vi "Finite Sound Input.vi"() -> ()   [LabVIEW 2023]
doc: "This VI illustrates how to acquire a finite number of samples from a specified device. It requires the use of a microphone attached to the sound card. You can specify the number of samples to acquire, sample rate, number of channels and a bit rate per sample."
uses:
  <vilib>/sound2/lvsound2.llb/Sampling Mode.ctl
  <vilib>/sound2/lvsound2.llb/Sound Data Format.ctl
  <vilib>/sound2/lvsound2.llb/Sound Input Read (DBL).vi
panel:
  in  "Device ID":u32
  out "Sound Input":waveform(dbl)[](graph)
  in  "Number of Samples/ch":i32=10000
  # "Overview: Demonstrates the use of the Sound Functions to acquire a finite number of samples from a microphone attached to the sound card.\nRequirements: Microphone\nInstructions:\n1. Specify the Device ID and Number of Samples/ch.\n2. Run the VI."
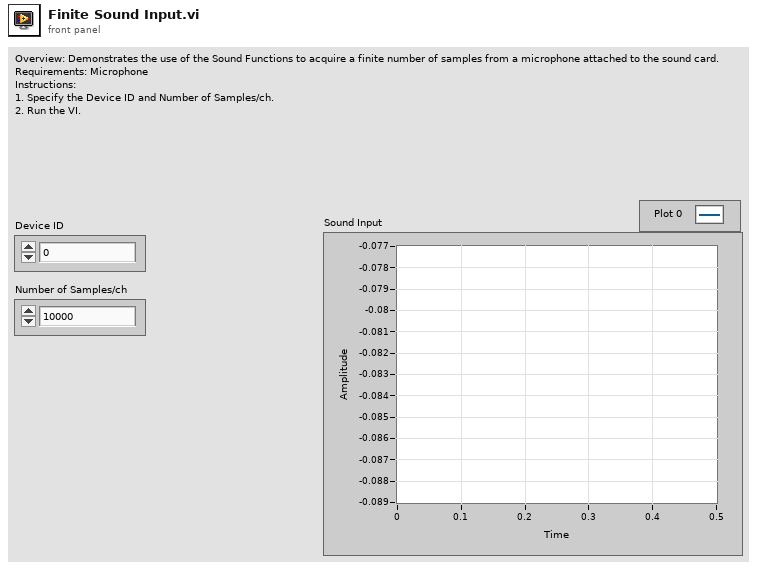
[diagram p1: front panel]
types:
  T1 = typedef "Sound Data Format.ctl" = cluster{"sample rate (S/s)":dbl, "number of channels":i32, "bits per sample":i32}
  T2 = typedef "Sampling Mode.ctl" = i32
  T3 = typedef "Sound Input Task ID.ctl" = u32
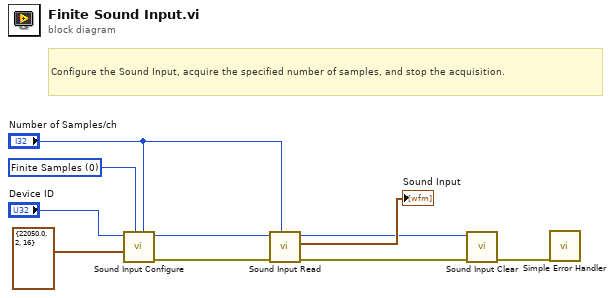
[diagram p0: block diagram]
diagram:
  w6 = T2 0 items=["Finite Samples", "Continuous Samples"] ("sample mode")
  # "Configure the Sound Input, acquire the specified number of samples, and stop the acquisition."
  n1 = call <vilib>:"Sound Input Configure.vi"("number of samples/ch"="Number of Samples/ch", "sample mode"=w6, "sound format"=T1 {"sample rate (S/s)"=22050.0, "number of channels"=2, "bits per sample"=16} ("Sound Format"), "device ID"="Device ID") -> ("error out"=w9:errorcluster, "task ID"=w7:T3)  [unwired: 6 in]
  n2 = call-poly <vilib>:"Sound Input Read.vi"("number of samples/ch"="Number of Samples/ch", "error in (no error)"=w9, "task ID"=w7) -> ("error out"=w4:errorcluster, "data"=→"Sound Input":waveform(dbl)[], "task ID out"=w5:T3)  [unwired: 6 in]
  n3 = call <vilib>:"Sound Input Clear.vi"("error in (no error)"=w4, "task ID"=w5) -> ("error out"=w1:errorcluster)  [unwired: 9 in]
  n4 = call <vilib>:"Simple Error Handler.vi"("error in (no error)"=w1) -> ()  [unwired: 4 in, 5 out]
